vi "Initialize Packet.vi"(8 "error in (no error)":errorcluster, 10 "Protocol Version":i32, 11 "Packet A in":refnum<class "Packet A.lvclass">) -> (0 "error out":errorcluster, 3 "Packet A out":refnum<class "Packet A.lvclass">)   [LabVIEW 2019, in "Packet A.lvclass"]
uses:
  Packet A.lvclass
  Packet A.lvclass/Packet A.ctl
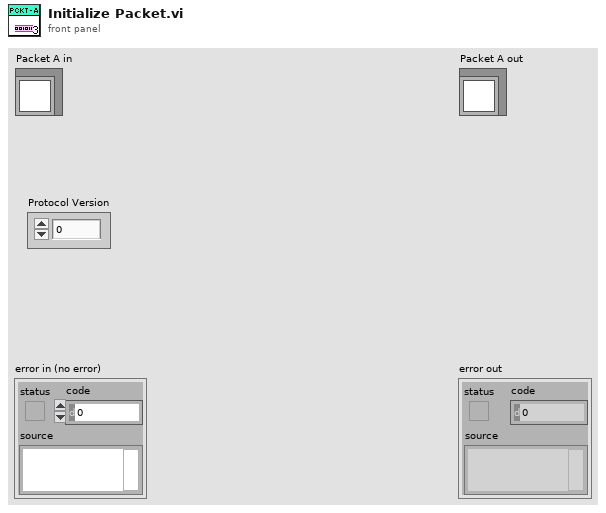
[diagram p1: front panel]
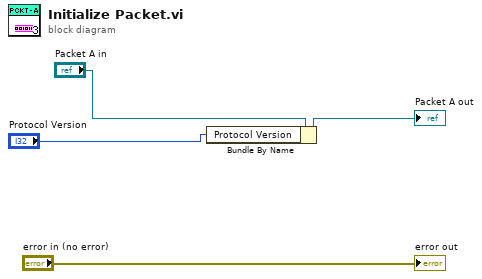
[diagram p0: block diagram]
diagram:
  n1 = Bundle By Name(cluster="Packet A in", "Protocol Version"="Protocol Version") -> (→"Packet A out":refnum<class "Packet A.lvclass">)
  "error out" <- "error in (no error)"
